vi "Set Manual Mode.vi"(8 "error in (no error)":errorcluster, 9 "Power":dbl, 10 "Manual Mode":bool, 11 "Temp Control in":refnum<class "Temp Control.lvclass">) -> (0 "error out":errorcluster, 3 "Temp Control out":refnum<class "Temp Control.lvclass">)   [LabVIEW 2022 SP3, in "Temp Control.lvclass"]
uses:
  Temp Control.lvclass
  Temp Control.lvclass/Temp Control.ctl
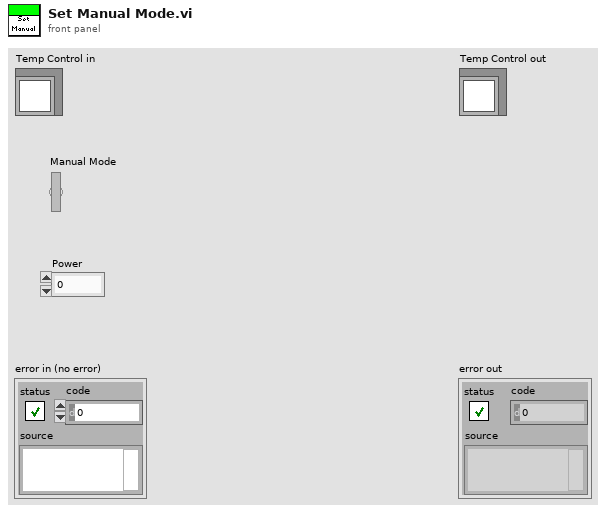
[diagram p1: front panel]
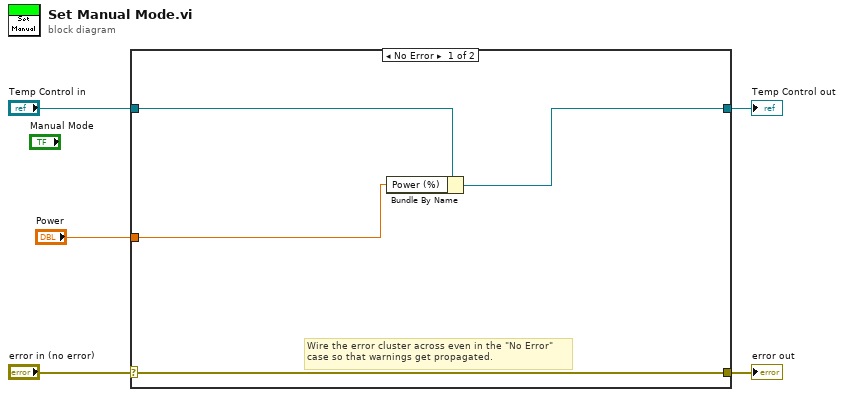
[diagram p0: block diagram]
diagram:
  n1 = case shown="No Error" "error in (no error)" {
    selector: "error in (no error)" -> [w9 w11]
    tunnel: [w9 w11] -> w4
    tunnel: [w7 w10] -> w2
    tunnel: "Temp Control in" -> [w6 w10]
    tunnel: "Power" -> [w8 _]
    frame No Error {
      # "Wire the error cluster across even in the \"No Error\"\ncase so that warnings get propagated."
      n2 = Bundle By Name(cluster=w6, "Power (%)"=w8) -> (w7:refnum<class "Temp Control.lvclass">)
    }
    frame Error {
    }
  }
  "error out" <- w4
  "Temp Control out" <- w2
